vi "BuildDataNumeric.vi"(9 "new element/subarray":dbl, 11 "element":dbl) -> (2 "[0]":dbl)   [LabVIEW 2011]
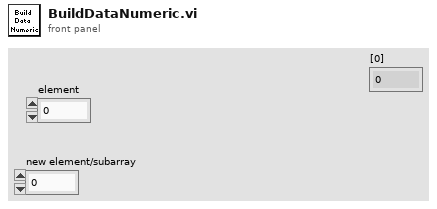
[diagram p1: front panel]
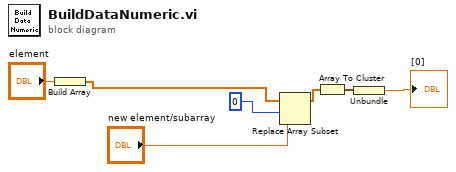
[diagram p0: block diagram]
diagram:
  n1 = Build Array("element") -> (w7:dbl[])
  n2 = Replace Array Subset(array=w7, new element="new element/subarray", index=0) -> (w4:dbl[])
  n3 = Array To Cluster(array=w4) -> (cluster=w6:cluster{"[0]":dbl})
  n4 = Unbundle(w6) -> ("[0]"=→"[0]":dbl)
